vi "ScanWaveforms.vi"() -> ()   [LabVIEW 2016]
uses:
  controls/ScanWaveform.ctl
  controls/Enum.ctl
  Course Project/support/Message Queue/Message Cluster.ctl
  <vilib>/rvi/errors/niLvFpgaAdjustHostInterfaceError.vi
  <vilib>/Utility/file.llb/Read Delimited Spreadsheet (DBL).vi
  controls/FPGAVIreferenceTypeDefScanEngine.ctl
  <vilib>/rvi/interface/nirviReadWriteControl/nirviReadWriteControl.xnode
  FPGA Bitfiles/qnmController797_usbRio80MHz_1.lvbitx
  <vilib>/regexp/Match Regular Expression.xnode
  Course Project/support/Message Queue/Message Queue.lvlib
  NiFpgaLv.dll
panel:
  in  "scanWaveFormCtl":T2={"slowWavePts"=1024, "fastWavePts"=1024, "slowWaveType"=enum."Triangle", "fastWaveType"=enum."Rounded", "slowRoundPts"=8, "fastRoundPts"=32, "Update Parameters"=FALSE, "UpdateFPGA"=FALSE, "Update Graph"=FALSE, "Hysteresis comp?"=FALSE, "Hysteresis"=FALSE, "Resonance"=FALSE, "Resonance comp?"=FALSE, "Hyst Source"=enum."Config"}
  in  "ScanWaveform":enum32{"ScanWaveform"}(tab)
  out "Waveforms":waveform(dbl)[](graph)
  # "Update"
  # "Parameters"
  # "Compensate"
  # "Fast"
  # "Slow"
  # "Nb of points"
  # "Rounding"
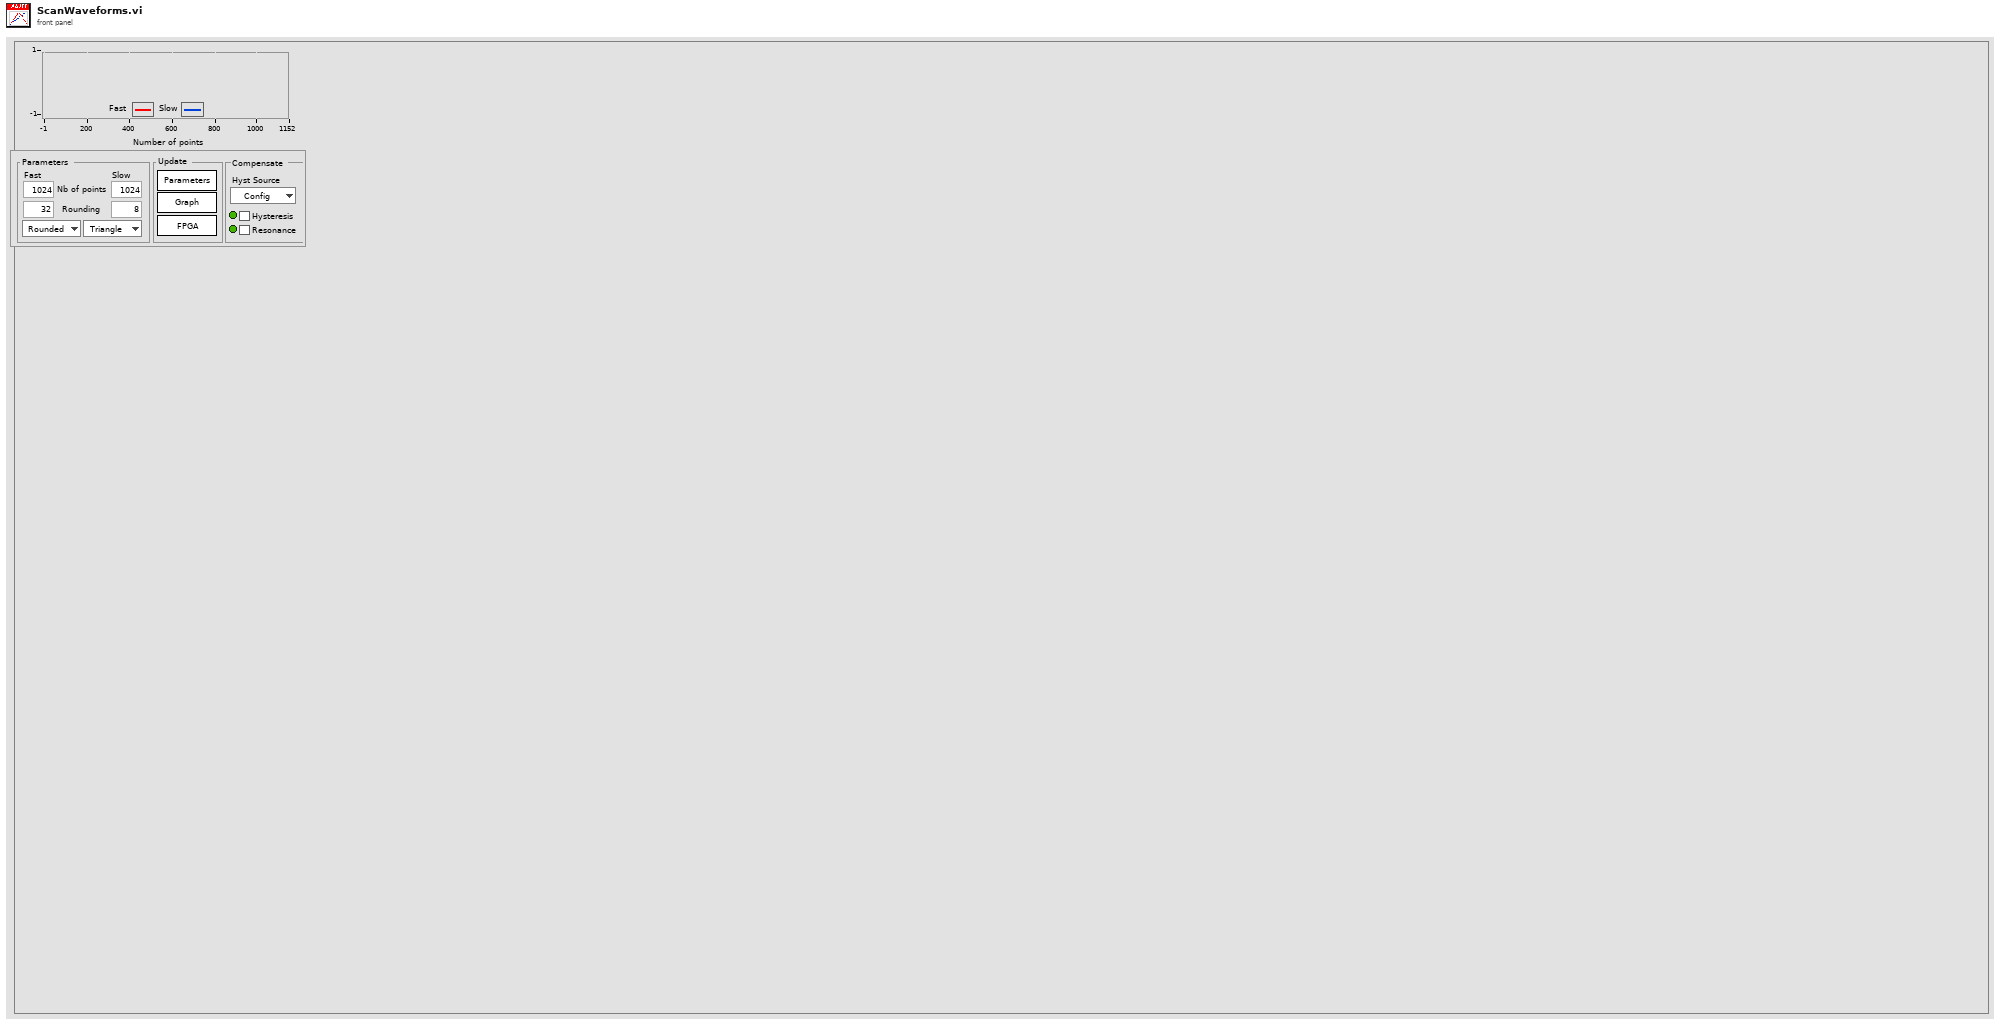
[diagram p1: front panel]
types:
  T1 = typedef "ScanWaveform.ctl" = enum16{"Sine", "Triangle", "Rounded"}
  T2 = cluster{"slowWavePts":u16, "fastWavePts":u16, "slowWaveType":T1, "fastWaveType":T1, "slowRoundPts":u16, "fastRoundPts":u16, "Update Parameters":bool, "UpdateFPGA":bool, "Update Graph":bool, "Hysteresis comp?":bool, "Hysteresis":bool, "Resonance":bool, "Resonance comp?":bool, "Hyst Source":enum16{"Config", "Scan"}}
  T3 = typedef "Message Queue.lvlib/All Message Queues.ctl" = cluster{"IU":refnum<queue>}
  T4 = typedef "Enum.ctl" = enum16{"Init", "Read", "Write"}
  T5 = typedef "Message Queue.lvlib/Message Cluster.ctl" = cluster{"Message":string, "Données de message":variant}
  T6 = typedef "FPGAVIreferenceTypeDefScanEngine.ctl" = refnum<k20>
  T7 = cluster{"CorrectionToFGV":bool, "PolynomCoeff":dbl[], "CorrectionToFPGA":bool}
  T8 = cluster{"slowWavePts":u16, "fastWavePts":u16, "slowWaveType":T1, "fastWaveType":T1, "slowRoundPts":u16, "fastRoundPts":u16, "singleDirectionScan":bool}
  T9 = cluster{"startFwd":u16, "endFwd":u16, "startBwd":u16, "endBwd":u16, "disableBlanking":bool, "useFineCounter":bool}
  T10 = cluster{"outputRate":u16, "fastDecFactor":u16, "outWaveSizeFast":u16, "pplUpsampling":u16, "numLines":u16, "se.p.fastInvDec":fxp<+,22,0>, "se.p.slowUpStep":fxp<+,28,0>, "se.p.outWaveSizeSlow":u16, "blankingMax":u32, "se.p.fastBlanking":cluster{"startFwd":u32, "endFwd":u32, "startBwd":u32, "endBwd":u32, "disableBlanking":bool, "useCoarseCounter":bool}}
  T11 = cluster{"Waveform Shape Fast In":dbl[], "Waveform Shape Slow In":dbl[]}
  T12 = cluster{"write":bool, "index":u16, "data":fxp<+/-,18,5>}
  T13 = cluster{"se.p.enable":bool, "se.p.singleDirection":bool, "se.p.haltScan":bool, "se.mot.p.start":bool}
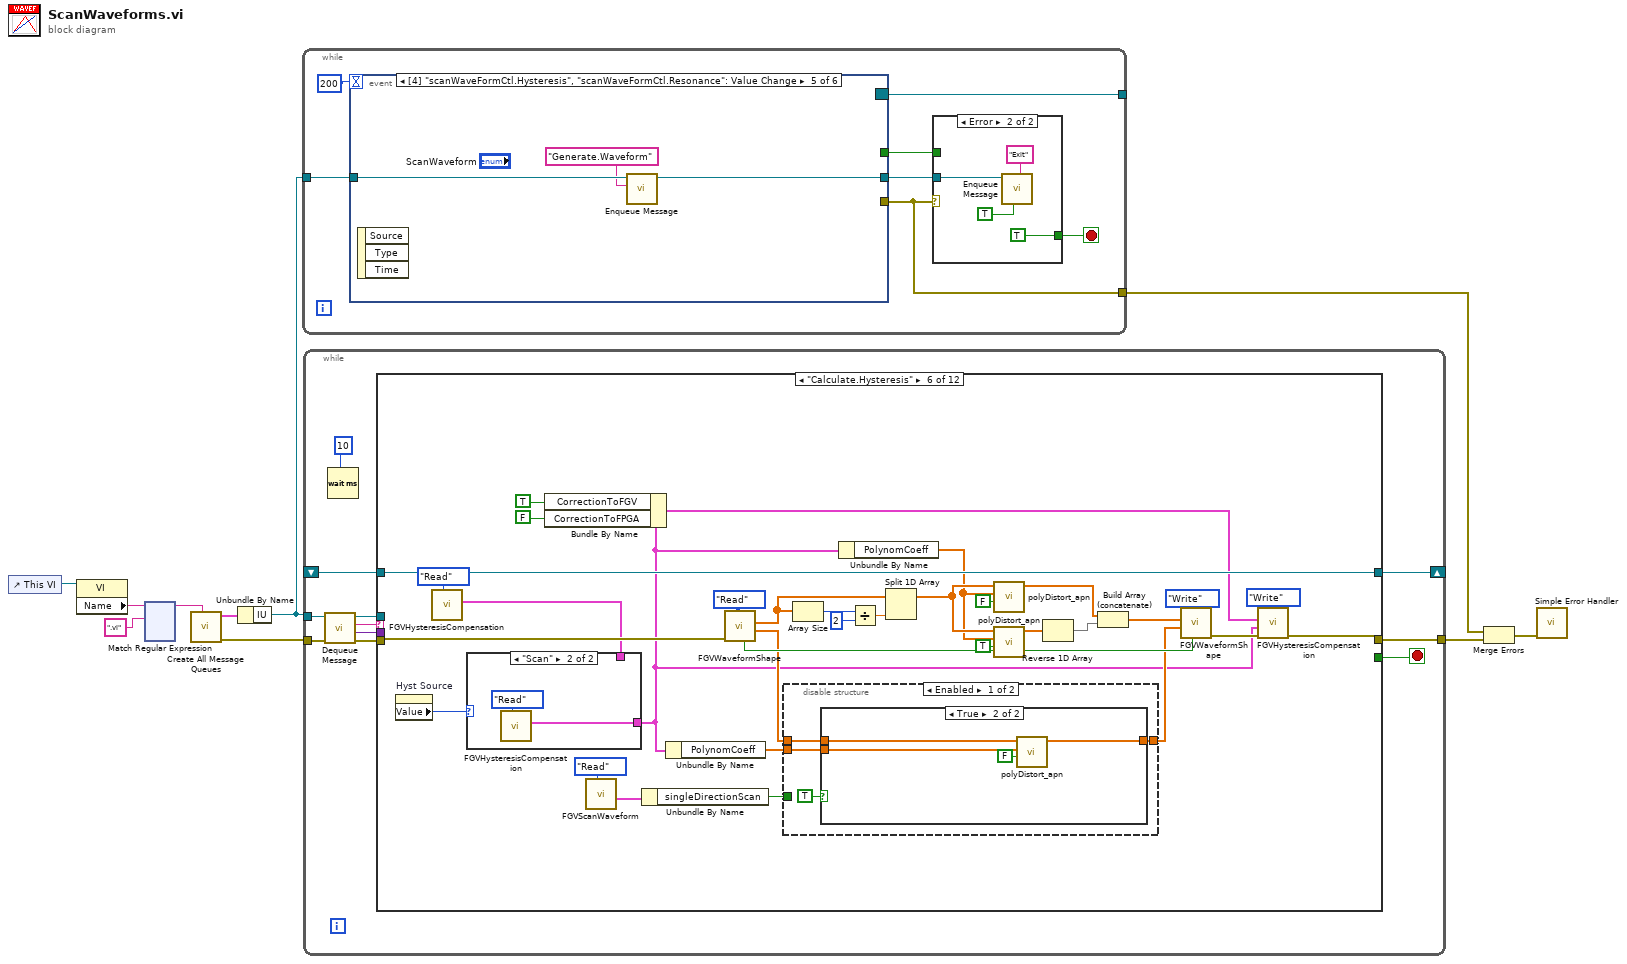
[diagram p0: block diagram]
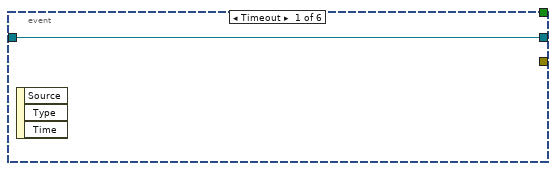
[diagram p3: hidden frame]
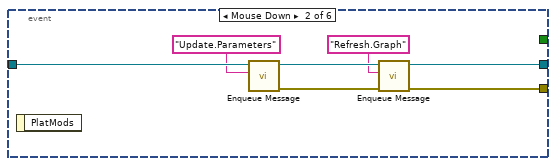
[diagram p4: hidden frame]
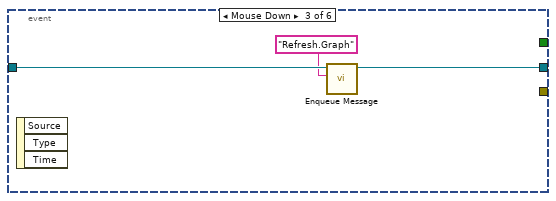
[diagram p5: hidden frame]
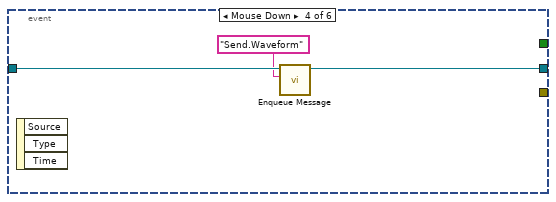
[diagram p6: hidden frame]
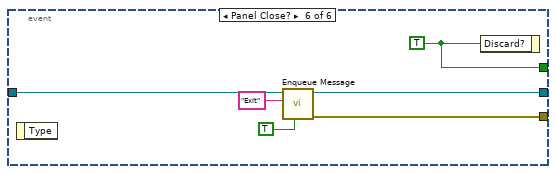
[diagram p7: hidden frame]
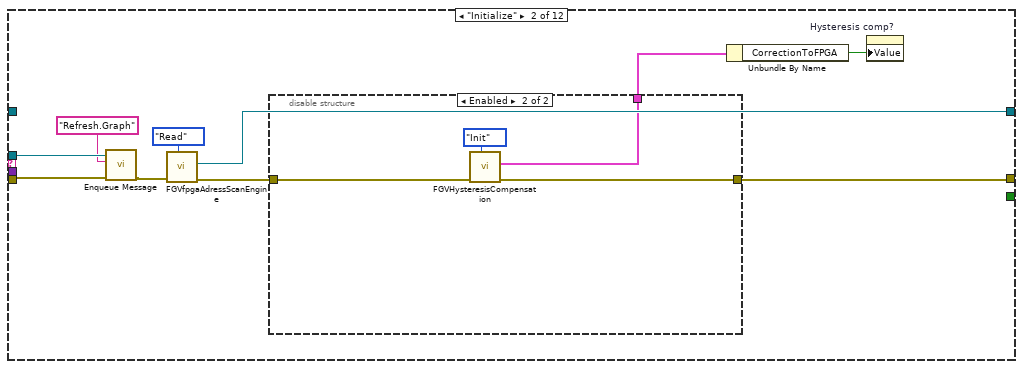
[diagram p9: hidden frame]
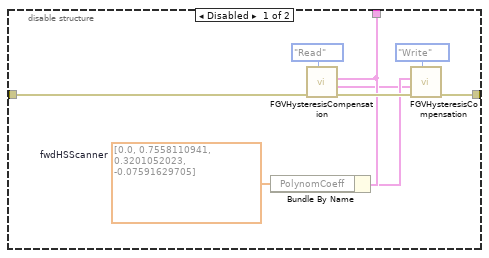
[diagram p10: hidden frame]
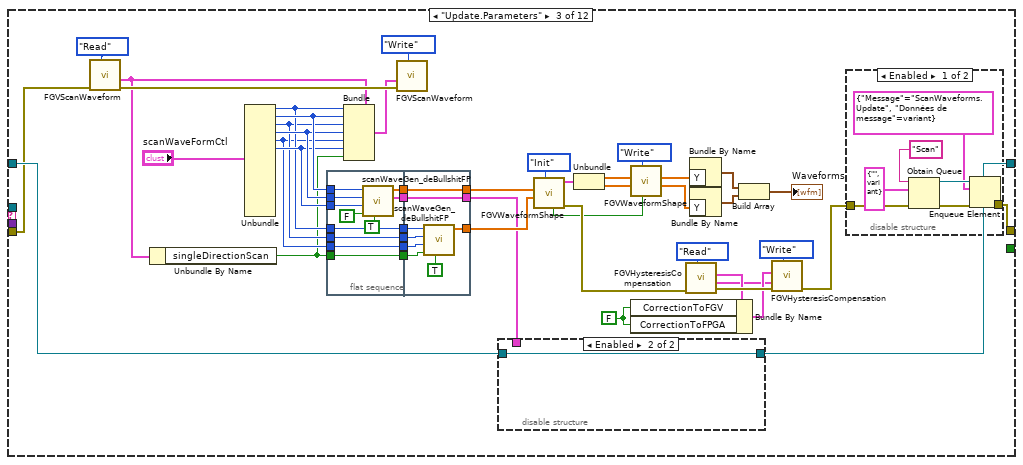
[diagram p11: hidden frame]
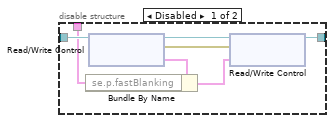
[diagram p13: hidden frame]
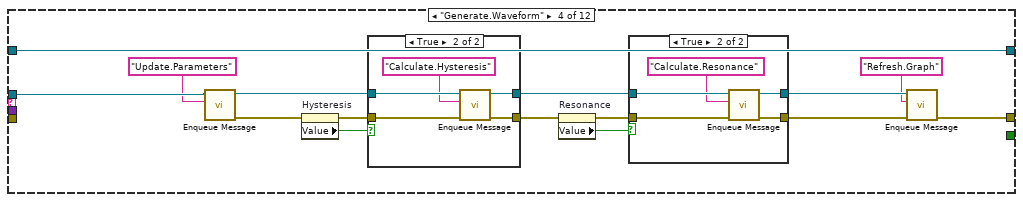
[diagram p14: hidden frame]
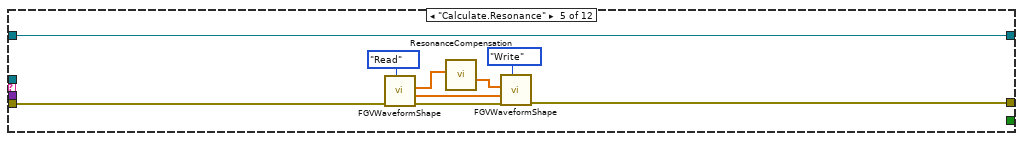
[diagram p17: hidden frame]
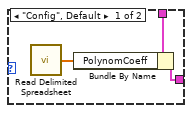
[diagram p18: hidden frame]
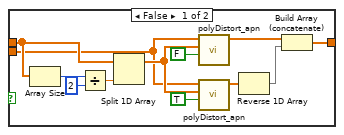
[diagram p19: hidden frame]
diagram:
  n1 = control-ref of="This VI"() -> (w4:refnum<vi>)
  n2 = property class="VI"(reference=w4) -> ("Name"=w3:string)  [unwired: 1 in, 2 out]
  n3 = xnode "Match Regular Expression"("input string"=w3, "regular expression"=".vi") -> ("before match"=w1:string)  [unwired: 4 in, 4 out]
  n4 = call "Create All Message Queues.vi"("QueueName"=w1) -> ("ErrorOut"=w8:errorcluster, "MessageQueueOut"=w10:T3)  [unwired: 9 in]
  n5 = Unbundle By Name(w10) -> ("IU"=w9:refnum<queue>)
  n6 = while {
    tunnel: w9 -> [w17]
    tunnel: [w13] -> w5
    tunnel: [w12] -> _
    stop <- w15 stop-if-true
    n7 = event shown="[4] \"scanWaveFormCtl.Hysteresis\", \"scanWaveFormCtl.Resonance\": Value Change" {
      selector: _ -> [_ _ _ _ _ _]
      dyn-events: [_ _ _ _ _ _] -> w12
      timeout: 200 -> [_ _ _ _ _ _]
      tunnel: [_ _ _ _ _ w45] -> w16
      tunnel: w17 -> [w23 w29 w33 w36 w39 w44]
      tunnel: [_ w25 _ _ _ w43] -> w13
      tunnel: [w23 w24 w32 w35 w38 w42] -> w14
      event Timeout {
        n8 = event-data() -> ()  [unwired: 1 in, 3 out]
      }
      event "scanWaveFormCtl.Update Parameters": Mouse Down {
        n9 = event-data() -> ()  [unwired: 1 in, 1 out]
        n10 = call "Enqueue Message.vi"("Message"="Update.Parameters", "Queue"=w29) -> ("error out"=w26:errorcluster, "Queue dup."=w30:refnum<queue>)  [unwired: 8 in]
        n11 = call "Enqueue Message.vi"("error in"=w26, "Message"="Refresh.Graph", "Queue"=w30) -> ("error out"=w25:errorcluster, "Queue dup."=w24:refnum<queue>)  [unwired: 7 in]
      }
      event "scanWaveFormCtl.Update Graph": Mouse Down {
        n12 = event-data() -> ()  [unwired: 1 in, 3 out]
        n13 = call "Enqueue Message.vi"("Message"="Refresh.Graph", "Queue"=w33) -> ("Queue dup."=w32:refnum<queue>)  [unwired: 8 in, 1 out]
      }
      event "scanWaveFormCtl.UpdateFPGA": Mouse Down {
        n14 = event-data() -> ()  [unwired: 1 in, 3 out]
        n15 = call "Enqueue Message.vi"("Message"="Send.Waveform", "Queue"=w36) -> ("Queue dup."=w35:refnum<queue>)  [unwired: 8 in, 1 out]
      }
      event "scanWaveFormCtl.Hysteresis", "scanWaveFormCtl.Resonance": Value Change {
        n16 = event-data() -> ()  [unwired: 1 in, 3 out]
        n17 = call "Enqueue Message.vi"("Message"="Generate.Waveform", "Queue"=w39) -> ("Queue dup."=w38:refnum<queue>)  [unwired: 8 in, 1 out]
      }
      event Panel Close? {
        w45 = TRUE ("Rejeter ?")
        n18 = event-data() -> ()  [unwired: 1 in, 1 out]
        n19 = call "Enqueue Message.vi"("Prioritary message"=TRUE ("Message prioritaire ? (F)"), "Message"="Exit", "Queue"=w44) -> ("error out"=w43:errorcluster, "Queue dup."=w42:refnum<queue>)  [unwired: 7 in]
        n20 = event-data ("Event Filter Node")("Discard?"=w45) -> ()  [unwired: 1 in, 1 out]
      }
    }
    n21 = case shown="Error" w13 {
      tunnel: [w18 TRUE ("Rejeter ?")] -> w15
      tunnel: w16 -> [w18 _]
      tunnel: w14 -> [_ w21]
      frame No Error {
      }
      frame Error {
        n22 = call "Enqueue Message.vi"("Prioritary message"=TRUE ("Message prioritaire ? (F)"), "Message"="Exit", "Queue"=w21) -> ()  [unwired: 7 in, 2 out]
      }
    }
  }
  n23 = while {
    tunnel: w9 -> [w50]
    tunnel: w8 -> [w54]
    tunnel: [w55] -> w6
    shift-right: [w48] -> _
    shift-left: _ -> [w47]
    stop <- w56 stop-if-true
    n24 = call "Dequeue Message.vi"("entrée d'erreur (pas d'erreur)"=w54, "File d'attente de messages"=w50) -> ("sortie d'erreur"=w53:errorcluster, "Données de message"=w52:variant, "Message"=w49:string, "File d'attente de message dup."=w51:refnum<queue>)  [unwired: 6 in]
    n25 = Wait (ms)(milliseconds to wait=u32 10 ("millisecond timer value")) -> ()  [unwired: 1 out]
    n26 = case "Conditions des messages" shown="\"Calculate.Hysteresis\"" w49 {
      selector: w49 -> [_ _ _ _ _ _ _ _ _ _ _ w350]
      tunnel: w51 -> [_ w68 _ w176 _ _ _ _ w321 _ w345 _]
      tunnel: w53 -> [w57 w60 w85 _ w193 w221 w268 w315 w318 w334 w343 _]
      tunnel: [w57 w62 w84 w169 w194 w222 w267 w315 w319 w334 w342 w348] -> w55
      tunnel: [_ _ _ _ _ _ _ _ _ _ TRUE _] -> w56
      tunnel: w52 -> [_ _ _ _ _ _ _ _ _ _ _ _]
      tunnel: [w58 w67 w86 w175 w200 w233 w275 w314 w320 w333 w341 w346] -> w48
      tunnel: w47 -> [w58 _ w125 w175 w200 w233 w274 w314 w320 w333 w341 w346]
      frame "--------- Initialization ---------" {
      }
      frame "Initialize" {
        n27 = call "Enqueue Message.vi"("error in"=w60, "Message"="Refresh.Graph", "Queue"=w68) -> ("error out"=w59:errorcluster)  [unwired: 7 in, 1 out]
        n28 = call "FGVfpgaAdressScanEngine.vi"("Enum"=Enum."Read", "error in"=w59) -> ("error out"=w63:errorcluster, "FPGA.SEout"=w67:T6)  [unwired: 5 in, 3 out]
        n29 = disable-structure shown="Enabled" {
          disable-tunnel: [w75 w78] -> w64
          disable-tunnel: w63 -> [w73 w80]
          disable-tunnel: [w72 w79] -> w62
          frame Disabled {
            w70 = dbl[] [0.0, 0.7558110941, 0.3201052023, -0.07591629705]  # fwdHSScanner
            n30 = call "FGVHysteresisCompensation.vi"("Enum"=Enum."Read", "error in"=w73) -> ("error out"=w77:errorcluster, "HysteresisSlowOut"=w69:T7, "HysteresisFastOut"=w75:T7)  [unwired: 7 in]
            n31 = Bundle By Name(cluster=w75, "PolynomCoeff"=w70) -> (w74:T7)
            n32 = call "FGVHysteresisCompensation.vi"("Enum"=Enum."Write", "error in"=w77, "HysteresisSlowIn"=w69, "HysteresisFastIn"=w74) -> ("error out"=w72:errorcluster)  [unwired: 5 in, 2 out]
          }
          frame Enabled {
            n33 = call "FGVHysteresisCompensation.vi"("Enum"=Enum."Init", "error in"=w80) -> ("error out"=w79:errorcluster, "HysteresisFastOut"=w78:T7)  [unwired: 7 in, 1 out]
          }
        }
        n34 = Unbundle By Name(w64) -> ("CorrectionToFPGA"=w65:bool)
        n35 = property on="Hysteresis comp?" class="Bool (strict)"("Value"=w65) -> ()  [unwired: 2 in, 2 out]
      }
      frame "Update.Parameters" {
        w96 = FALSE ("Correction?")
        n36 = call "FGVScanWaveform.vi"("Enum"=Enum."Read", "error in"=w85) -> ("error out"=w127:errorcluster, "scanWaveFormCtl Out"=w112:T8)  [unwired: 8 in]
        n37 = Unbundle By Name(w112) -> ("singleDirectionScan"=w105:bool)
        n38 = Unbundle("scanWaveFormCtl") -> ("slowWavePts"=w108:u16, "fastWavePts"=w111:u16, "slowWaveType"=w107:T1, "fastWaveType"=w110:T1, "slowRoundPts"=w106:u16, "fastRoundPts"=w109:u16)  [unwired: 8 out]
        n39 = flat-sequence {
          tunnel: w111 -> [w154]
          tunnel: w110 -> [w153]
          tunnel: w109 -> [w152]
          tunnel: [w150] -> w124
          tunnel: w108 -> [w150]
          tunnel: w107 -> [w149]
          tunnel: [w149] -> w123
          tunnel: [w148] -> w122
          tunnel: w106 -> [w148]
          tunnel: w105 -> [w147]
          tunnel: [w147] -> w121
          tunnel: [w146] -> w120
          tunnel: [w145] -> w119
          tunnel: w124 -> [w157]
          tunnel: w123 -> [w162]
          tunnel: w122 -> [w161]
          tunnel: w121 -> [w160]
          tunnel: w120 -> [w159]
          tunnel: [w159] -> w104
          tunnel: [w158] -> w103
          tunnel: w119 -> [w156]
          tunnel: [w156] -> w102
          frame #0 {
            n40 = call "scanWaveGen_deBullshitFP.vi"("overScanBlanking"=TRUE, "singleDirScan"=FALSE, "numRoundingPts"=w152, "scanWaveForm"=w153, "numPts"=w154) -> ("blankingParams"=w145:T9, "outWave"=w146:dbl[])  [unwired: 5 in]
          }
          frame #1 {
            n41 = call "scanWaveGen_deBullshitFP.vi"("overScanBlanking"=TRUE, "singleDirScan"=w160, "numRoundingPts"=w161, "scanWaveForm"=w162, "numPts"=w157) -> ("outWave"=w158:dbl[])  [unwired: 5 in, 1 out]
          }
        }
        n42 = Bundle(cluster=w112, "slowWavePts"=w108, "fastWavePts"=w111, "slowWaveType"=w107, "fastWaveType"=w110, "slowRoundPts"=w106, "fastRoundPts"=w109, "singleDirectionScan"=w105) -> (w114:T8)
        n43 = call "FGVScanWaveform.vi"("Enum"=Enum."Write", "error in"=w127, "scanWaveFormCtl In"=w114) -> ()  [unwired: 7 in, 2 out]
        n44 = disable-structure shown="Enabled" {
          disable-tunnel: w125 -> [w142 w143]
          disable-tunnel: w102 -> [w141 _]
          disable-tunnel: [w137 w143] -> w86
          frame Disabled {
            n45 = xnode "Read/Write Control"("FPGA VI Reference In"=w142) -> ("FPGA VI Reference Out"=w136:T6, "error out"=w140:errorcluster, "se.p.clocks"=w139:T10)  [unwired: 1 in]
            n46 = Bundle By Name(cluster=w139, "se.p.fastBlanking"=w141) -> (w138:T10)
            n47 = xnode "Read/Write Control"("FPGA VI Reference In"=w136, "error in"=w140, "se.p.clocks"=w138) -> ("FPGA VI Reference Out"=w137:T6)  [unwired: 1 out]
          }
          frame Enabled {
          }
        }
        n48 = call "FGVWaveformShape.vi"("Enum"=Enum."Init", "Waveform Shape Slow In"=w103, "Waveform Shape Fast In"=w104) -> ("error out"=w95:errorcluster, "WaveformInit"=w101:T11, "Framing up? (down: f) out"=w89:bool)  [unwired: 4 in, 2 out]
        n49 = Unbundle(w101) -> ("Waveform Shape Fast In"=w93:dbl[], "Waveform Shape Slow In"=w91:dbl[])
        n50 = call "FGVWaveformShape.vi"("Framing up? (down: f) In"=w89, "Enum"=Enum."Write", "Waveform Shape Slow In"=w91, "Waveform Shape Fast In"=w93) -> ("Waveform Shape Slow Out"=w90:dbl[], "Waveform Shape Fast Out"=w92:dbl[])  [unwired: 3 in, 3 out]
        n51 = call "FGVHysteresisCompensation.vi"("Enum"=Enum."Read", "error in"=w95) -> ("error out"=w126:errorcluster, "HysteresisSlowOut"=w82:T7, "HysteresisFastOut"=w98:T7)  [unwired: 7 in]
        n52 = Bundle By Name(cluster=w98, "CorrectionToFGV"=w96, "CorrectionToFPGA"=w96) -> (w97:T7)
        n53 = Bundle By Name("Y"=w92) -> (w117:waveform(dbl))  [unwired: 1 in]
        n54 = Bundle By Name("Y"=w90) -> (w118:waveform(dbl))  [unwired: 1 in]
        n55 = Build Array(w117, w118) -> (→"Waveforms":waveform(dbl)[])
        n56 = call "FGVHysteresisCompensation.vi"("Enum"=Enum."Write", "error in"=w126, "HysteresisSlowIn"=w82, "HysteresisFastIn"=w97) -> ("error out"=w83:errorcluster)  [unwired: 5 in, 2 out]
        n57 = disable-structure shown="Enabled" {
          disable-tunnel: [w129 w135] -> w84
          disable-tunnel: w83 -> [w128 w135]
          frame Enabled {
            n58 = Obtain Queue(name (unnamed)="Scan", element data type=T5 {"Message"="", "Données de message"=variant} ("Cluster Message"), error in (no error)=w128) -> (queue out=w133:refnum<queue>, error out=w132:errorcluster)  [unwired: 2 in, 1 out]
            n59 = Enqueue Element(queue=w133, element=T5 {"Message"="ScanWaveforms.Update", "Données de message"=variant} ("Cluster Message"), error in (no error)=w132) -> (error out=w129:errorcluster)  [unwired: 1 in, 2 out]
          }
          frame Disabled {
          }
        }
      }
      frame "Generate.Waveform" {
        n60 = call "Enqueue Message.vi"("Message"="Update.Parameters", "Queue"=w176) -> ("error out"=w166:errorcluster, "Queue dup."=w167:refnum<queue>)  [unwired: 8 in]
        n61 = property on="Hysteresis" class="Bool (strict)"(error in=w166) -> (error out=w173:errorcluster, "Value"=w171:bool)  [unwired: 1 in, 1 out]
        n62 = case shown="True" w171 {
          tunnel: w167 -> [w178 w184]
          tunnel: [w179 w182] -> w165
          tunnel: w173 -> [w179 w181]
          tunnel: [w178 w180] -> w164
          frame False {
          }
          frame True {
            n63 = call "Enqueue Message.vi"("error in"=w181, "Message"="Calculate.Hysteresis", "Queue"=w184) -> ("error out"=w182:errorcluster, "Queue dup."=w180:refnum<queue>)  [unwired: 7 in]
          }
        }
        n64 = property on="Resonance" class="Bool (strict)"(error in=w165) -> (error out=w168:errorcluster, "Value"=w172:bool)  [unwired: 1 in, 1 out]
        n65 = case shown="True" w172 {
          tunnel: [w186 w191] -> w177
          tunnel: w164 -> [w186 w190]
          tunnel: [w185 w188] -> w163
          tunnel: w168 -> [w185 w187]
          frame False {
          }
          frame True {
            n66 = call "Enqueue Message.vi"("error in"=w187, "Message"="Calculate.Resonance", "Queue"=w190) -> ("error out"=w188:errorcluster, "Queue dup."=w191:refnum<queue>)  [unwired: 7 in]
          }
        }
        n67 = call "Enqueue Message.vi"("error in"=w163, "Message"="Refresh.Graph", "Queue"=w177) -> ("error out"=w169:errorcluster)  [unwired: 7 in, 1 out]
      }
      frame "Calculate.Resonance" {
        n68 = call "FGVWaveformShape.vi"("Enum"=Enum."Read", "error in"=w193) -> ("error out"=w192:errorcluster, "Waveform Shape Slow Out"=w197:dbl[], "Waveform Shape Fast Out"=w199:dbl[])  [unwired: 5 in, 2 out]
        n69 = call "ResonanceCompensation.vi"("Waveform Shape Fast Out"=w199) -> ("CorrectedWaveform"=w198:dbl[])  [unwired: 8 in, 2 out]
        n70 = call "FGVWaveformShape.vi"("Enum"=Enum."Write", "error in"=w192, "Waveform Shape Slow In"=w197, "Waveform Shape Fast In"=w198) -> ("error out"=w194:errorcluster)  [unwired: 3 in, 4 out]
      }
      frame "Calculate.Hysteresis" {
        n71 = property on="Hyst Source" class="Enum (strict)"() -> ("Value"=w203:enum16{"Config", "Scan"})  [unwired: 2 in, 2 out]
        n72 = call "FGVHysteresisCompensation.vi"("Enum"=Enum."Read") -> ("HysteresisFastOut"=w201:T7)  [unwired: 8 in, 2 out]
        n73 = case shown="\"Scan\"" w203 {
          tunnel: [w234 w237] -> w206
          tunnel: w201 -> [w236 _]
          frame "Config", Default {
            n74 = call-poly <vilib>:"Read Delimited Spreadsheet.vi"() -> ("first row"=w235:dbl[])  [unwired: 10 in, 5 out]
            n75 = Bundle By Name(cluster=w236, "PolynomCoeff"=w235) -> (w234:T7)
          }
          frame "Scan" {
            n76 = call "FGVHysteresisCompensation.vi"("Enum"=Enum."Read") -> ("HysteresisFastOut"=w237:T7)  [unwired: 8 in, 2 out]
          }
        }
        n77 = Bundle By Name(cluster=w206, "CorrectionToFGV"=TRUE ("Correction?"), "CorrectionToFPGA"=FALSE) -> (w227:T7)
        n78 = call "FGVScanWaveform.vi"("Enum"=Enum."Read") -> ("scanWaveFormCtl Out"=w225:T8)  [unwired: 9 in, 1 out]
        n79 = Unbundle By Name(w225) -> ("singleDirectionScan"=w217:bool)
        n80 = Unbundle By Name(w206) -> ("PolynomCoeff"=w205:dbl[])
        n81 = call "FGVWaveformShape.vi"("Enum"=Enum."Read", "error in"=w221) -> ("Waveform Shape Slow Out"=w209:dbl[], "Waveform Shape Fast Out"=w210:dbl[], "Framing up? (down: f) out"=w230:bool)  [unwired: 5 in, 2 out]
        n82 = disable-structure shown="Enabled" {
          disable-tunnel: w217 -> [_ _]
          disable-tunnel: [w242 w259] -> w207
          disable-tunnel: w209 -> [w241 w259]
          disable-tunnel: w205 -> [w240 _]
          frame Enabled {
            n83 = case shown="True" TRUE {
              tunnel: [w249 w256] -> w242
              tunnel: w241 -> [w244 w257]
              tunnel: w240 -> [w243 w255]
              frame False {
                n84 = Array Size(array=w244) -> (size(s)=w247:i32)
                n85 = Divide(x=w247, y=2) -> (x/y=w248:dbl)
                n86 = Split 1D Array(array=w244, index=w248) -> (first subarray=w245:dbl[])  [unwired: 1 out]
                n87 = call "polyDistort_apn.vi"("Backward?"=FALSE, "polyIn"=w245, "lineDataIn"=w243) -> ("distoredDataOut"=w251:dbl[])  [unwired: 7 in, 1 out]
                n88 = call "polyDistort_apn.vi"("Backward?"=TRUE, "polyIn"=w245, "lineDataIn"=w243) -> ("distoredDataOut"=w252:dbl[])  [unwired: 7 in, 1 out]
                n89 = Reverse 1D Array(array=w252) -> (reversed array=w250:dbl[])
                n90 = Build Array (concatenate)(w251, w250) -> (w249:dbl[])
              }
              frame True {
                n91 = call "polyDistort_apn.vi"("Backward?"=FALSE, "polyIn"=w255, "lineDataIn"=w257) -> ("distoredDataOut"=w256:dbl[])  [unwired: 7 in, 1 out]
              }
            }
          }
          frame Disabled {
          }
        }
        n92 = Array Size(array=w210) -> (size(s)=w214:i32)
        n93 = Unbundle By Name(w206) -> ("PolynomCoeff"=w204:dbl[])
        n94 = Divide(x=w214, y=2) -> (x/y=w213:dbl)
        n95 = Split 1D Array(array=w210, index=w213) -> (first subarray=w211:dbl[])  [unwired: 1 out]
        n96 = call "polyDistort_apn.vi"("Backward?"=FALSE, "polyIn"=w204, "lineDataIn"=w211) -> ("distoredDataOut"=w208:dbl[])  [unwired: 7 in, 1 out]
        n97 = call "polyDistort_apn.vi"("Backward?"=TRUE, "polyIn"=w204, "lineDataIn"=w211) -> ("distoredDataOut"=w218:dbl[])  [unwired: 7 in, 1 out]
        n98 = Reverse 1D Array(array=w218) -> (reversed array=w216:dbl[])
        n99 = Build Array (concatenate)(w208, w216) -> (w212:dbl[])
        n100 = call "FGVWaveformShape.vi"("Framing up? (down: f) In"=w230, "Enum"=Enum."Write", "Waveform Shape Slow In"=w207, "Waveform Shape Fast In"=w212) -> ("error out"=w232:errorcluster)  [unwired: 3 in, 4 out]
        n101 = call "FGVHysteresisCompensation.vi"("Enum"=Enum."Write", "error in"=w232, "HysteresisSlowIn"=w206, "HysteresisFastIn"=w227) -> ("error out"=w222:errorcluster)  [unwired: 5 in, 2 out]
      }
      frame "Send.Waveform" {
        w269 = T12 {"write"=TRUE, "index"=0, "data"=0.0} ("slowWaveWrite")
        w271 = T12 {"write"=FALSE, "index"=0, "data"=0.0} ("fastWaveWrite")
        # "Send the Waveform, point by point, to the FPGA."
        n102 = xnode "Read/Write Control"("FPGA VI Reference In"=w274, "error in"=w268) -> ("FPGA VI Reference Out"=w289:T6, "error out"=w290:errorcluster, "se.p.modes"=w291:T13)
        n103 = Bundle By Name(cluster=w291, "se.p.enable"=FALSE ("scanEnabled")) -> (w292:T13)
        n104 = xnode "Read/Write Control"("FPGA VI Reference In"=w289, "error in"=w290, "se.p.modes"=w292) -> ("FPGA VI Reference Out"=w297:T6, "error out"=w266:errorcluster)
        n105 = call "FGVHysteresisCompensation.vi"("Enum"=Enum."Read") -> ("HysteresisSlowOut"=w260:T7, "HysteresisFastOut"=w278:T7)  [unwired: 8 in, 1 out]
        n106 = call "FGVWaveformShape.vi"("Enum"=Enum."Read", "error in"=w266) -> ("Waveform Shape Slow Out"=w296:dbl[], "Waveform Shape Fast Out"=w295:dbl[])  [unwired: 5 in, 3 out]
        n107 = Unbundle By Name(w278) -> ("CorrectionToFGV"=w280:bool)
        n108 = for {
          tunnel: [w304] -> w288
          tunnel: w296 -> [w303] mode=indexing
          tunnel: w269 -> [w299]
          tunnel: w297 -> [w302]
          tunnel: [w305] -> w287
          i -> [w298]
          n109 = To Fixed-Point(number=w303) -> (fixed-point=w300:fxp<+/-,18,5>)  [unwired: 1 in]
          n110 = Bundle By Name(cluster=w299, "data"=w300, "index"=w298) -> (w301:T12)
          n111 = xnode "Read/Write Control"("FPGA VI Reference In"=w302, "se.m.slowAxis"=w301) -> ("FPGA VI Reference Out"=w305:T6, "error out"=w304:errorcluster)  [unwired: 1 in]
        }
        n112 = for {
          tunnel: [w312] -> w286
          tunnel: w295 -> [w311] mode=indexing
          tunnel: w269 -> [w307]
          tunnel: w297 -> [w310]
          tunnel: [w313] -> w285
          i -> [w306]
          n113 = To Fixed-Point(number=w311) -> (fixed-point=w308:fxp<+/-,18,5>)  [unwired: 1 in]
          n114 = Bundle By Name(cluster=w307, "data"=w308, "index"=w306) -> (w309:T12)
          n115 = xnode "Read/Write Control"("FPGA VI Reference In"=w310, "se.m.fastAxis"=w309) -> ("FPGA VI Reference Out"=w313:T6, "error out"=w312:errorcluster)  [unwired: 1 in]
        }
        n116 = Equal?(x=w280, y=TRUE) -> (x = y?=w273:bool)
        n117 = Bundle By Name(cluster=w278, "CorrectionToFPGA"=w273) -> (w277:T7)
        n118 = xnode "Read/Write Control"("FPGA VI Reference In"=w285, "error in"=w286, "se.m.fastAxis"=w271) -> ("FPGA VI Reference Out"=w275:T6, "error out"=w284:errorcluster)
        n119 = xnode "Read/Write Control"("FPGA VI Reference In"=w287, "error in"=w288, "se.m.slowAxis"=w271) -> ("error out"=w283:errorcluster)  [unwired: 1 out]
        n120 = Merge Errors(w284, w283) -> (w272:errorcluster)
        n121 = call "FGVHysteresisCompensation.vi"("Enum"=Enum."Write", "error in"=w272, "HysteresisSlowIn"=w260, "HysteresisFastIn"=w277) -> ("error out"=w270:errorcluster)  [unwired: 5 in, 2 out]
        n122 = property on="UpdateFPGA" class="Bool (strict)"(error in=w270, "Value"=FALSE) -> (error out=w261:errorcluster)  [unwired: 1 in, 1 out]
        n123 = property on="Hysteresis" class="Bool (strict)"(error in=w261) -> (error out=w263:errorcluster, "Value"=w264:bool)  [unwired: 1 in, 1 out]
        n124 = property on="Resonance" class="Bool (strict)"(error in=w261) -> (error out=w262:errorcluster, "Value"=w265:bool)  [unwired: 1 in, 1 out]
        n125 = property on="Hysteresis comp?" class="Bool (strict)"(error in=w263, "Value"=w264) -> (error out=w267:errorcluster)  [unwired: 1 in, 1 out]
        n126 = property on="Resonance comp?" class="Bool (strict)"(error in=w262, "Value"=w265) -> ()  [unwired: 1 in, 2 out]
      }
      frame "------- From Other VIs -------" {
      }
      frame "Speed.Update" {
        n127 = property on="Resonance" class="Bool (strict)"(error in=w318) -> (error out=w317:errorcluster, "Value"=w316:bool)  [unwired: 1 in, 1 out]
        n128 = case shown="True" w316 {
          tunnel: w321 -> [_ w326]
          tunnel: [w322 w324] -> w319
          tunnel: w317 -> [w322 w323]
          frame False {
          }
          frame True {
            n129 = call "Enqueue Message.vi"("error in"=w323, "Message"="Generate.Waveform", "Queue"=w326) -> ("error out"=w324:errorcluster)  [unwired: 7 in, 1 out]
          }
        }
      }
      frame "Refresh.Graph" {
        n130 = call "FGVWaveformShape.vi"("Enum"=Enum."Read") -> ("Waveform Shape Slow Out"=w327:dbl[], "Waveform Shape Fast Out"=w328:dbl[])  [unwired: 6 in, 3 out]
        n131 = disable-structure shown="Enabled" {
          disable-tunnel: w328 -> [w340 _]
          disable-tunnel: w327 -> [w339 _]
          frame Enabled {
            n132 = Array Size(array=w339) -> (size(s)=w338:i32)
            n133 = Array Size(array=w340) -> (size(s)=w337:i32)
            n134 = Max & Min(x=w338, y=w337) -> (max(x,y)=w336:i32)  [unwired: 1 out]
            n135 = To Double Precision Float(number=w336) -> (double precision float=w335:dbl)
            n136 = property on="Waveforms" class="WFGraph (strict)"("XScale.Maximum"=w335) -> ()  [unwired: 2 in, 2 out]
          }
          frame Disabled {
          }
        }
        n137 = Bundle By Name("Y"=w328) -> (w330:waveform(dbl))  [unwired: 1 in]
        n138 = Bundle By Name("Y"=w327) -> (w331:waveform(dbl))  [unwired: 1 in]
        n139 = Build Array(w330, w331) -> (w332:waveform(dbl)[])
        n140 = local write "Waveforms"(w332) -> ()
      }
      frame "Exit" {
        n141 = Release Queue(queue=w345, error in (no error)=w343) -> (error out=w342:errorcluster)  [unwired: 1 in, 2 out]
      }
      frame Default {
        n142 = Format Into String(format string="The message\"%s\" received in the gestion loop is not valid" ("Texte de message d'erreur inconnu"), w350) -> (resulting string=w347:string)  [unwired: 2 in, 1 out]
        n143 = call <vilib>:"Error Cluster From Error Code.vi"("error message (\"\")"=w347, "error code (0)"=1 ("code d'erreur (0)")) -> ("error out"=w348:errorcluster)  [unwired: 7 in]
      }
    }
  }
  n144 = Merge Errors(w5, w6) -> (w7:errorcluster)
  n145 = call <vilib>:"Simple Error Handler.vi"("error in (no error)"=w7) -> ()  [unwired: 4 in, 5 out]
